vi "spot_gen_ver2.vi"(0 "amp":u32, 5 "input valid":bool, 7 "data index":u16, 9 "peak":bool, 11 "reciver_params":T1) -> (4 "PDW":u64, 6 "output valid":bool, 15 "timieng":bool)   [LabVIEW 2021]
uses:
  reciver params.ctl
  <vilib>/rvi/Memory/Memory_Emulation/nirvimemoryFastEmulation.vi
  <vilib>/rvi/Memory/Memory_Emulation/nirvimemoryEmulation.vi
  <vilib>/rvi/Emulation/niFpgaEmulationIsFPGAContextNoSignature.vi
  <vilib>/rvi/DataTransferAndStorage/Container/Common/niFpgaContainerGetUniqueNameForEmu.vi
  <vilib>/rvi/Emulation/niFpgaProcessEmulError.vi
  <vilib>/rvi/Emulation/niFpgaSctlEmulationGetInTimedLoop.vi
  <vilib>/rvi/errors/nirviReportUnexpectedCaseInternalError (U32).vi
  <vilib>/rvi/FXPMathLib/basic elements/FxpAddSub/XNode/nifxpmath_AddSub.xnode
  <vilib>/rvi/DataTransferAndStorage/Container/XNode/niFpgaContainer.xnode
  <vilib>/rvi/FXPMathLib/sim/FxpSim.dll
  <vilib>/rvi/FXPMathLib/FxpAdd/XNode/nifxpmath_Add.xnode
  <vilib>/rvi/FXPMathLib/FxpSub/XNode/nifxpmath_Sub.xnode
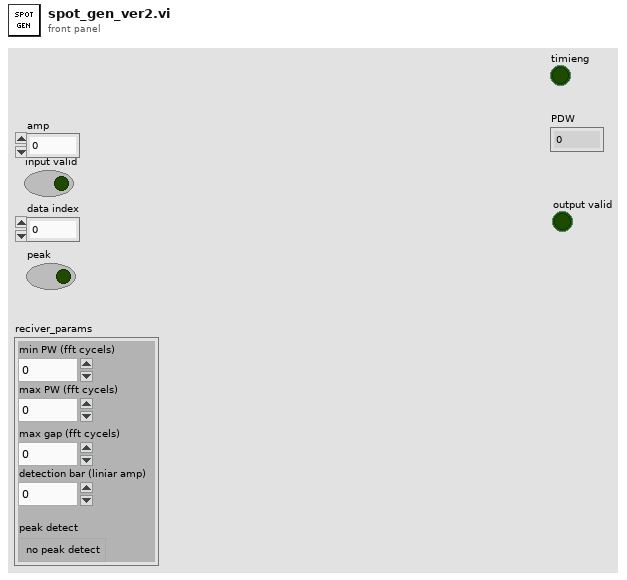
[diagram p1: front panel]
types:
  T1 = typedef "reciver params.ctl" = cluster{"min PW (fft cycels)":u16, "max PW (fft cycels)":u16, "max gap (fft cycels)":u8, "detection bar (liniar amp)":fxp<+,64,63>, "peak detect":bool}
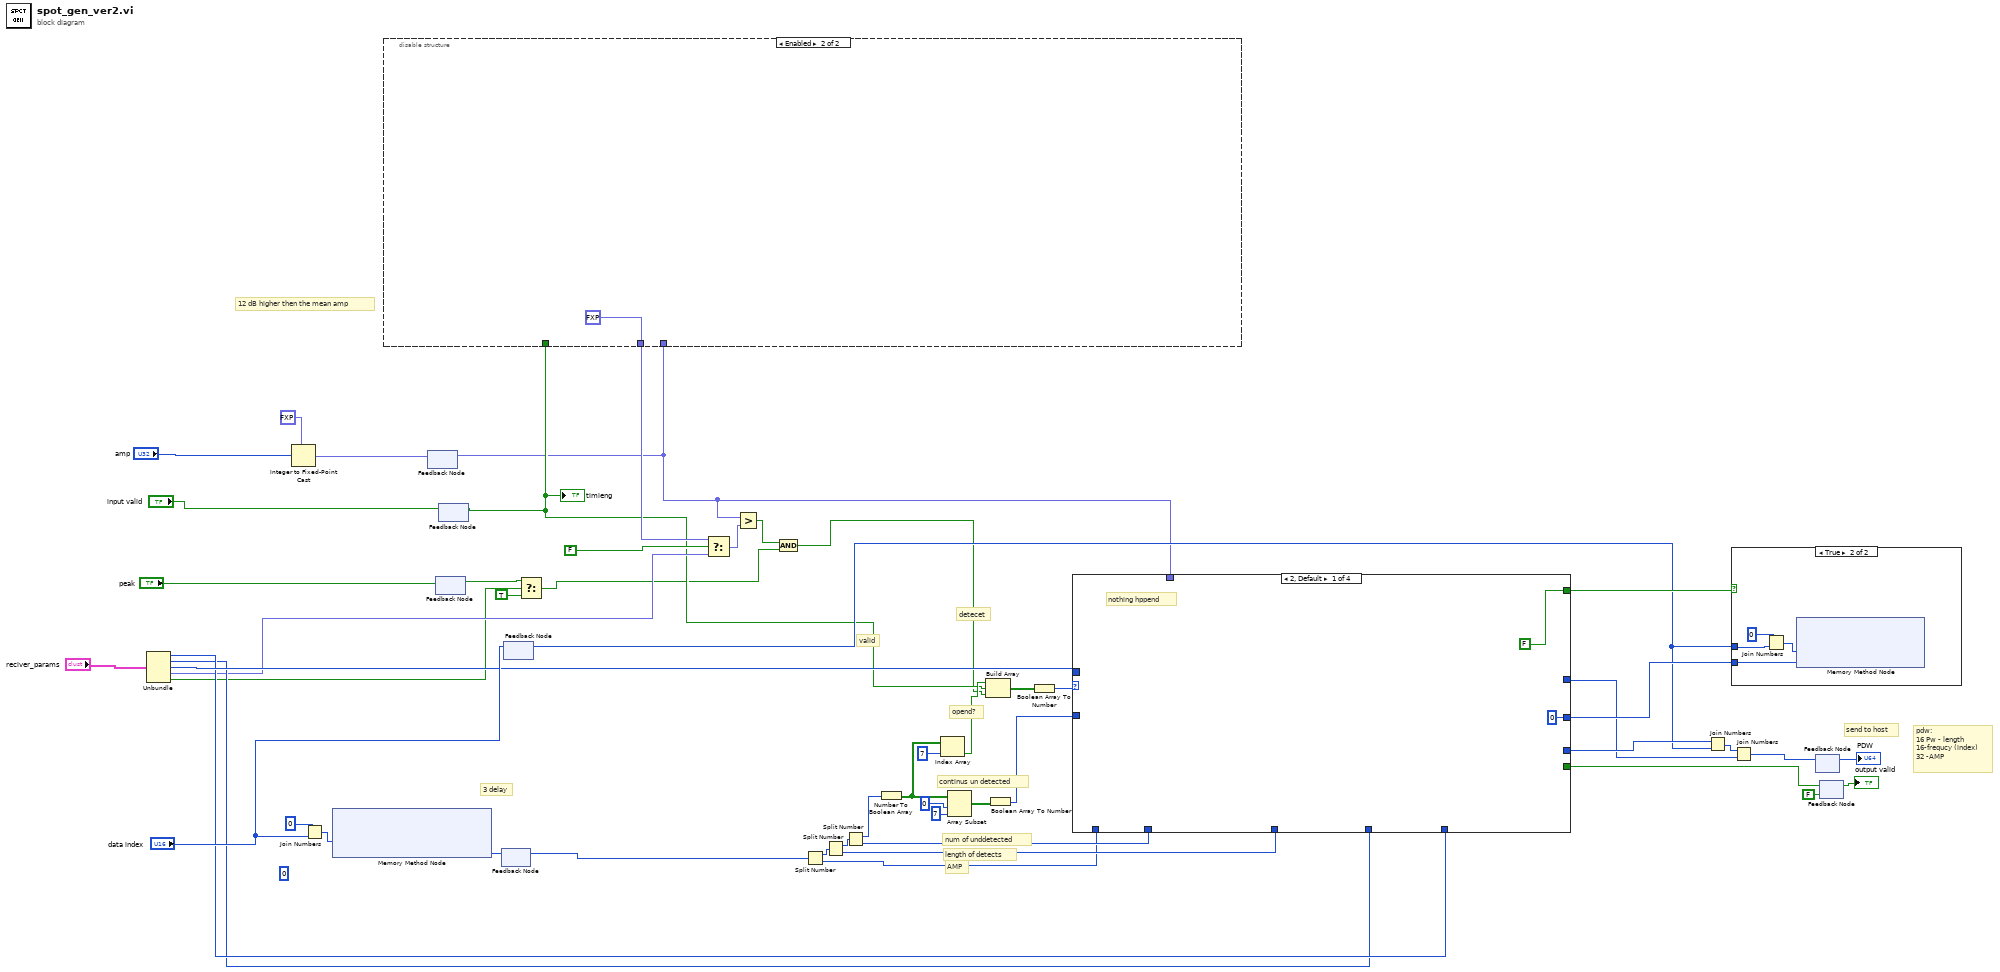
[diagram p0: block diagram]
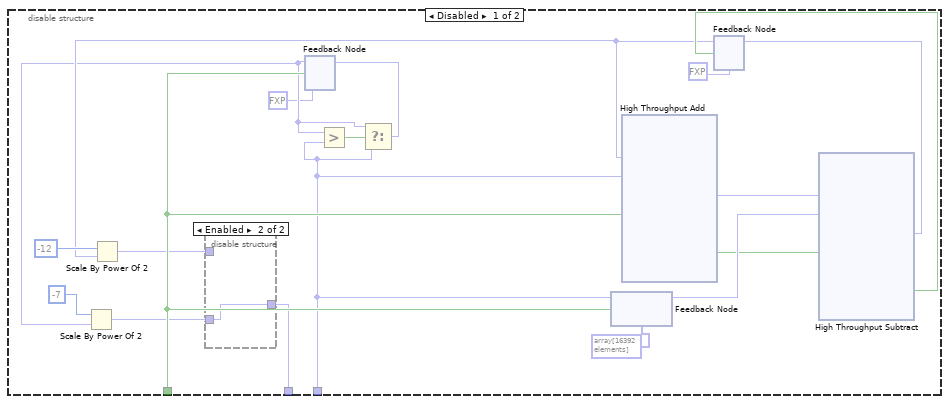
[diagram p2: hidden frame]
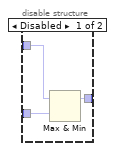
[diagram p3: hidden frame]
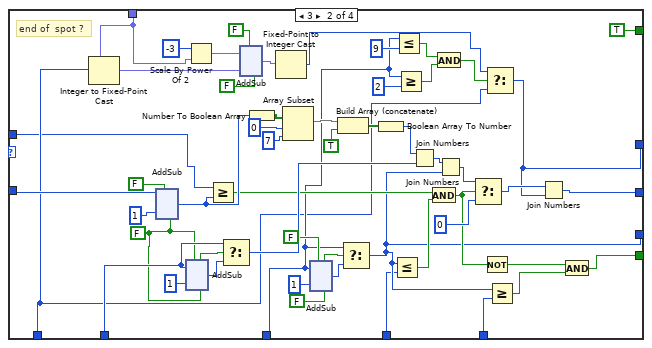
[diagram p5: hidden frame]
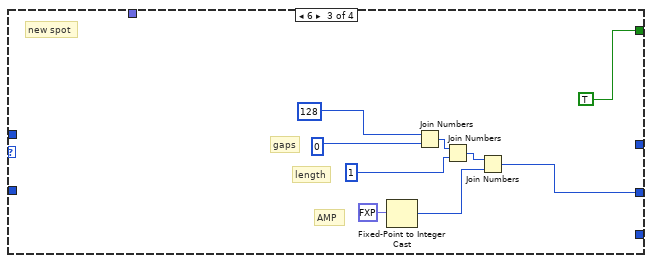
[diagram p6: hidden frame]
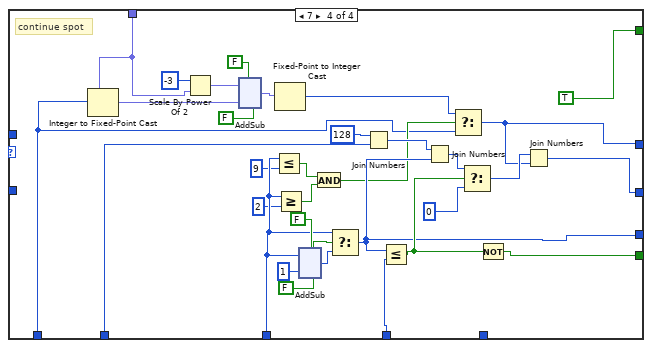
[diagram p7: hidden frame]
diagram:
  (unwired) u16 0 ("data index 2")
  # "12 dB higher then the mean amp"
  # "3 delay"
  # "AMP"
  # "pdw:\n16 Pw - length\n16-frequcy (index)\n32 -AMP"
  # "send to host"
  # "continus un detected"
  # "num of unddetected"
  # "length of detects"
  # "opend?"
  # "valid"
  # "detecet"
  n1 = Unbundle("reciver_params") -> ("min PW (fft cycels)"=w19:u16, "max PW (fft cycels)"=w18:u16, "max gap (fft cycels)"=w20:u8, "detection bar (liniar amp)"=w17:fxp<+,64,63>, "peak detect"=w1:bool)
  n2 = Integer to Fixed-Point Cast(fixed-point type=fxp<+,32,31> 0.0 ("magnitude"), integer="amp") -> (fixed-point=w6:fxp<+,32,31>)
  n3 = Join Numbers(hi=u16 0, lo="data index") -> ((hi.lo)=w24:u32)
  n4 = xnode ("Memory Method Node")("Address"=w24) -> ("Data"=w28:u64)  [unwired: 1 in, 1 out]
  n5 = feedback #1() -> (w10:fxp<+,32,31>)  [unwired: 1 in]
  n6 = feedback-in #1(w6) -> ()
  n7 = feedback #2() -> (w3:bool)  [unwired: 1 in]
  n8 = feedback-in #2("peak") -> ()
  n9 = feedback #3() -> (w11:bool)  [unwired: 1 in]
  "timieng" <- w11
  n10 = disable-structure shown="Enabled" {
    disable-tunnel: w11 -> [w63 _]
    disable-tunnel: [w57 fxp<+,32,31> 0.0 ("magnitude")] -> w14
    disable-tunnel: w10 -> [w53 _]
    frame Disabled {
      n11 = feedback #4(fxp<+,32,31> 0.0 ("magnitude")) -> (w58:fxp<+,32,31>)
      n12 = Scale By Power Of 2(n=i8 -7 ("x"), x=w58) -> (x*2^n=w56:fxp<+,32,31>)
      n13 = Greater?(x=w58, y=w53) -> (0:w62:bool)
      n14 = Select(t=w58, s=w62, f=w53) -> (s? t:f=w60:fxp<+,32,31>)
      n15 = feedback-in #4(w60, w63) -> ()
      n16 = feedback #5(fxp<+,32,31>[] array[16392 elements]) -> (w69:fxp<+,32,31>)
      n17 = feedback-in #5(w53, w63) -> ()
      n18 = feedback #6(fxp<+,32,31> 0.0 ("s")) -> (w61:fxp<+,47,46>)
      n19 = Scale By Power Of 2(n=i8 -12 ("x"), x=w61) -> (x*2^n=w55:fxp<+,47,46>)
      n20 = disable-structure shown="Enabled" {
        disable-tunnel: [w74 w75] -> w57
        disable-tunnel: w56 -> [w73 w75]
        disable-tunnel: w55 -> [w72 _]
        frame Disabled {
          n21 = Max & Min(x=w72, y=w73) -> (max(x,y)=w74:fxp<+,47,46>)  [unwired: 1 out]
        }
        frame Enabled {
        }
      }
      n22 = xnode "High Throughput Add"("x"=w61, "y"=w53, "input valid"=w63) -> ("x+y"=w68:fxp<+,47,46>, "output valid"=w64:bool)  [unwired: 1 in, 1 out]
      n23 = xnode "High Throughput Subtract"("x"=w68, "y"=w69, "input valid"=w64) -> ("x-y"=w67:fxp<+,47,46>, "output valid"=w65:bool)  [unwired: 1 in, 1 out]
      n24 = feedback-in #6(w67, w65) -> ()
    }
    frame Enabled {
    }
  }
  n25 = feedback-in #3("input valid") -> ()
  n26 = feedback #7() -> (w27:u64)  [unwired: 1 in]
  n27 = feedback-in #7(w28) -> ()
  n28 = feedback #8() -> (w30:u16)  [unwired: 1 in]
  n29 = feedback-in #8("data index") -> ()
  n30 = Select(t=w3, s=w1, f=TRUE) -> (s? t:f=w4:bool)
  n31 = Select(t=w14, s=FALSE, f=w17) -> (s? t:f=w15:fxp<+,64,63>)
  n32 = Greater?(x=w10, y=w15) -> (0:w9:bool)
  n33 = And(x=w9, y=w4) -> (x .and. y?=w8:bool)
  n34 = Split Number(x=w27) -> (hi(x)=w33:u32, lo(x)=w32:u32)
  n35 = Split Number(x=w33) -> (hi(x)=w52:u16, lo(x)=w43:u16)
  n36 = Split Number(x=w52) -> (hi(x)=w51:u8, lo(x)=w40:u8)
  n37 = Number To Boolean Array(number=w51) -> (Boolean array=w45:bool[])
  n38 = Index Array(array=w45, index=7) -> (element=w34:bool)
  n39 = Array Subset(array=w45, index=0, length=7) -> (w48:bool[])
  n40 = Build Array(w34, w11, w8) -> (w47:bool[])
  n41 = Boolean Array To Number(Boolean array=w48) -> (number=w42:u8)
  n42 = Boolean Array To Number(Boolean array=w47) -> (number=w46:u8)
  n43 = case shown="2, Default" w46 {
    tunnel: w43 -> [_ w86 _ w362]
    tunnel: w42 -> [_ w128 _ _]
    tunnel: [u64 0 ("Data") w98 w348 w366] -> w41
    tunnel: [FALSE TRUE TRUE TRUE] -> w39
    tunnel: w40 -> [_ w118 _ w381]
    tunnel: [_ w101 _ w375] -> w37
    tunnel: [_ w100 _ w374] -> w38
    tunnel: w32 -> [_ w83 _ w357]
    tunnel: w10 -> [_ w91 _ w369]
    tunnel: [_ w82 _ w355] -> w31
    tunnel: w20 -> [_ w81 _ _]
    tunnel: w19 -> [_ w80 _ _]
    tunnel: w18 -> [_ w79 _ w356]
    frame 2, Default {
      # "nothing hppend"
    }
    frame 3 {
      w107 = FALSE ("carry-in")
      # "end of  spot ?"
      n44 = Integer to Fixed-Point Cast(fixed-point type=w91, integer=w83) -> (fixed-point=w93:fxp<+,32,31>)
      n45 = xnode "AddSub"("x"=w128, "y"=u8 1, "carry-in"=w107, "use zero instead of x"=FALSE) -> ("s"=w129:u8)  [unwired: 1 out]
      n46 = Scale By Power Of 2(n=i16 -3, x=w91) -> (x*2^n=w94:fxp<+,32,31>)
      n47 = xnode "AddSub"("x"=w118, "y"=u8 1, "carry-in"=w107, "use zero instead of x"=w107) -> ("s"=w119:u8, "carry-out"=w120:bool)
      n48 = Greater Or Equal?(x=w81, y=w129) -> (x >= y?=w109:bool)
      n49 = Select(t=w118, s=w120, f=w119) -> (s? t:f=w117:u8)
      n50 = xnode "AddSub"("x"=w94, "y"=w93, "carry-in"=FALSE, "use zero instead of x"=FALSE) -> ("s"=w92:fxp<+,32,31>)  [unwired: 1 out]
      n51 = Number To Boolean Array(number=w129) -> (Boolean array=w125:bool[])
      n52 = Fixed-Point to Integer Cast(1:w92) -> (0:w84:u32)
      n53 = Array Subset(array=w125, index=0, length=7) -> (w104:bool[])
      n54 = xnode "AddSub"("x"=w86, "y"=u16 1, "carry-in"=FALSE, "use zero instead of x"=FALSE) -> ("s"=w114:u16, "carry-out"=w115:bool)
      n55 = Build Array (concatenate)(w104, TRUE) -> (w124:bool[])
      n56 = Select(t=w86, s=w115, f=w114) -> (s? t:f=w100:u16)
      n57 = Boolean Array To Number(Boolean array=w124) -> (number=w123:u8)
      n58 = Less Or Equal?(x=w100, y=w79) -> (x <= y?=w106:bool)
      n59 = Less Or Equal?(x=w86, y=u16 9) -> (x <= y?=w89:bool)
      n60 = Greater Or Equal?(x=w86, y=u16 2) -> (x >= y?=w90:bool)
      n61 = Join Numbers(hi=w123, lo=w117) -> ((hi.lo)=w130:u16)
      n62 = And(x=w109, y=w106) -> (x .and. y?=w108:bool)
      n63 = And(x=w89, y=w90) -> (x .and. y?=w85:bool)
      n64 = Join Numbers(hi=w130, lo=w100) -> ((hi.lo)=w113:u32)
      n65 = Select(t=w113, s=w108, f=u32 0 ("Data")) -> (s? t:f=w99:u32)
      n66 = Not(x=w108) -> (.not. x?=w103:bool)
      n67 = Select(t=w84, s=w85, f=w83) -> (s? t:f=w82:u32)
      n68 = Greater Or Equal?(x=w100, y=w80) -> (x >= y?=w102:bool)
      n69 = Join Numbers(hi=w99, lo=w82) -> ((hi.lo)=w98:u64)
      n70 = And(x=w103, y=w102) -> (x .and. y?=w101:bool)
    }
    frame 6 {
      # "gaps"
      # "length"
      # "AMP"
      # "new spot"
      n71 = Fixed-Point to Integer Cast(1:fxp<+,32,31> 0.0 ("fixed-point")) -> (0:w347:u32)
      n72 = Join Numbers(hi=u8 128, lo=u8 0 ("hi")) -> ((hi.lo)=w354:u16)
      n73 = Join Numbers(hi=w354, lo=u16 1 ("hi")) -> ((hi.lo)=w349:u32)
      n74 = Join Numbers(hi=w349, lo=w347) -> ((hi.lo)=w348:u64)
    }
    frame 7 {
      # "continue spot"
      n75 = Integer to Fixed-Point Cast(fixed-point type=w369, integer=w357) -> (fixed-point=w368:fxp<+,32,31>)
      n76 = Scale By Power Of 2(n=i16 -3, x=w369) -> (x*2^n=w370:fxp<+,32,31>)
      n77 = xnode "AddSub"("x"=w370, "y"=w368, "carry-in"=FALSE, "use zero instead of x"=FALSE) -> ("s"=w365:fxp<+,32,31>)  [unwired: 1 out]
      n78 = Less Or Equal?(x=w362, y=u16 9) -> (x <= y?=w363:bool)
      n79 = Fixed-Point to Integer Cast(1:w365) -> (0:w358:u32)
      n80 = Greater Or Equal?(x=w362, y=u16 2) -> (x >= y?=w364:bool)
      n81 = xnode "AddSub"("x"=w362, "y"=u16 1, "carry-in"=FALSE, "use zero instead of x"=FALSE) -> ("s"=w382:u16, "carry-out"=w383:bool)
      n82 = And(x=w363, y=w364) -> (x .and. y?=w359:bool)
      n83 = Select(t=w362, s=w383, f=w382) -> (s? t:f=w374:u16)
      n84 = Join Numbers(hi=u8 128, lo=w381) -> ((hi.lo)=w385:u16)
      n85 = Less Or Equal?(x=w374, y=w356) -> (x <= y?=w376:bool)
      n86 = Join Numbers(hi=w385, lo=w374) -> ((hi.lo)=w380:u32)
      n87 = Select(t=w358, s=w359, f=w357) -> (s? t:f=w355:u32)
      n88 = Select(t=w380, s=w376, f=u32 0 ("Data")) -> (s? t:f=w367:u32)
      n89 = Not(x=w376) -> (.not. x?=w375:bool)
      n90 = Join Numbers(hi=w367, lo=w355) -> ((hi.lo)=w366:u64)
    }
  }
  n91 = Join Numbers(hi=w38, lo=w30) -> ((hi.lo)=w36:u32)
  n92 = case shown="True" w39 {
    tunnel: w30 -> [_ w504]
    tunnel: w41 -> [_ w506]
    frame False {
    }
    frame True {
      n93 = Join Numbers(hi=u16 0, lo=w504) -> ((hi.lo)=w503:u32)
      n94 = xnode ("Memory Method Node")("Address"=w503, "Data"=w506) -> ()  [unwired: 1 in, 1 out]
    }
  }
  n95 = Join Numbers(hi=w36, lo=w31) -> ((hi.lo)=w23:u64)
  n96 = feedback #9() -> (→"PDW":u64)  [unwired: 1 in]
  n97 = feedback-in #9(w23) -> ()
  n98 = feedback #10(FALSE) -> (→"output valid":bool)
  n99 = feedback-in #10(w37) -> ()
